vi "Format Attribute.vi"(5 "Attribute Names":string[](array[string]), 6 "Indent":i32, 7 "Attribute Values":variant[](array[variant]), 11 "CAML in":refnum<class "CAML.lvclass">) -> (3 "CAML out":refnum<class "CAML.lvclass">, 4 "Attr Strings":string[](array[string]))   [LabVIEW 2020, in "CAML.lvlib" / "CAML.lvclass"]
uses:
  <vilib>/gpm_packages/@cs/persistence/source/CAML/CAML.lvclass
  <vilib>/gpm_packages/@cs/persistence/source/XML/XML.lvclass
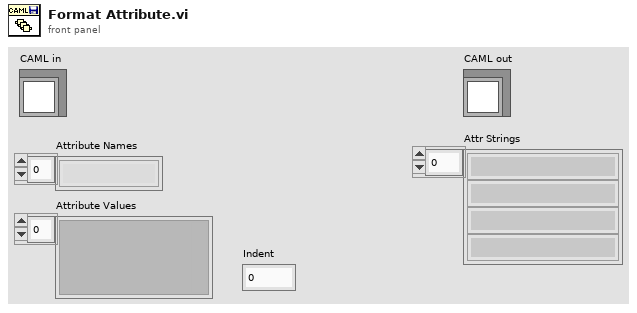
[diagram p1: front panel]
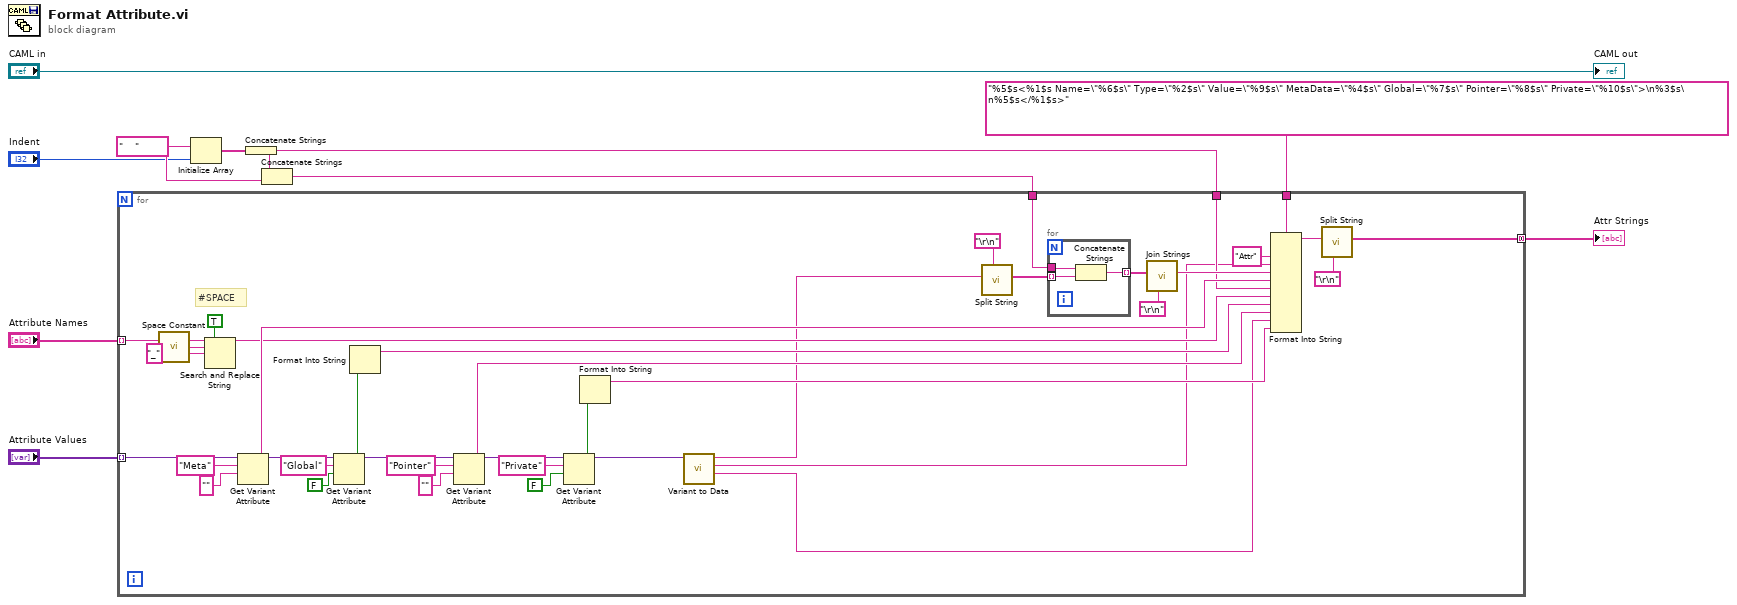
[diagram p0: block diagram]
diagram:
  w8 = "    "
  n1 = Initialize Array(w8, "Indent") -> (w9:string[])
  n2 = Concatenate Strings(w9) -> (w7:string)
  n3 = Concatenate Strings(w7, w8) -> (w5:string)
  n4 = for {
    tunnel: "Attribute Names" -> [w46] mode=indexing
    tunnel: "Attribute Values" -> [w44] mode=indexing
    tunnel: w7 -> [w28]
    tunnel: "%5$s<%1$s Name=\"%6$s\" Type=\"%2$s\" Value=\"%9$s\" MetaData=\"%4$s\" Global=\"%7$s\" Pointer=\"%8$s\" Private=\"%10$s\">\n%3$s\n%5$s</%1$s>" ("format string") -> [w36]
    tunnel: w5 -> [w33]
    tunnel: [w22] -> w1 mode=concatenating
    # "#SPACE"
    n5 = call <vilib>:"Space Constant.vi"() -> ("String"=w49:string)
    n6 = Search and Replace String(replace all?=TRUE ("replace all? (F)"), input string=w46, search string=w49, replace string="_") -> (result string=w27:string)  [unwired: 4 in, 3 out]
    n7 = Get Variant Attribute(Variant=w44, name="Meta", default value (empty Variant)="") -> (duplicate Variant=w43:variant, value=w29:string)  [unwired: 1 in, 2 out]
    n8 = Get Variant Attribute(Variant=w43, name="Global", default value (empty Variant)=FALSE) -> (duplicate Variant=w39:variant, value=w26:bool)  [unwired: 1 in, 2 out]
    n9 = Format Into String(w26) -> (resulting string=w25:string)  [unwired: 3 in, 1 out]
    n10 = Get Variant Attribute(Variant=w39, name="Pointer", default value (empty Variant)="") -> (duplicate Variant=w15:variant, value=w24:string)  [unwired: 1 in, 2 out]
    n11 = Get Variant Attribute(Variant=w15, name="Private", default value (empty Variant)=FALSE) -> (duplicate Variant=w14:variant, value=w17:bool)  [unwired: 1 in, 2 out]
    n12 = Format Into String(w17) -> (resulting string=w16:string)  [unwired: 3 in, 1 out]
    n13 = call <vilib>:"Variant to Data.vi"("Variant"=w14) -> ("String Value"=w11:string, "Type"=w12:string, "Value"=w13:string)  [unwired: 7 in, 1 out]
    n14 = call <vilib>:"Split String.vi"("Split Pattern"="\r\n", "Input String"=w13) -> ("Split String"=w34:string[])  [unwired: 9 in]
    n15 = for {
      tunnel: w34 -> [w52] mode=indexing
      tunnel: w33 -> [w51]
      tunnel: [w50] -> w32 mode=indexing
      n16 = Concatenate Strings(w51, w52) -> (w50:string)
    }
    n17 = call <vilib>:"Join Strings.vi"("Separator (,)"="\r\n", "Strings In"=w32) -> ("String"=w30:string)  [unwired: 9 in]
    n18 = Format Into String(format string=w36, "Attr" ("input 1"), w12, w30, w29, w28, w27, w25, w24, w11, w16) -> (resulting string=w23:string)  [unwired: 2 in, 1 out]
    n19 = call <vilib>:"Split String.vi"("Split Pattern"="\r\n", "Input String"=w23) -> ("Split String"=w22:string[])  [unwired: 9 in]
  }
  "Attr Strings" <- w1
  "CAML out" <- "CAML in"
